vi "lxc.vi"() -> ()   [LabVIEW 2017]
uses:
  <vilib>/Instr/_visa.llb/VISA Flush IO Buffer Mask.ctl
  <vilib>/Instr/_visa.llb/VISA Configure Serial Port (Instr).vi
panel:
  out "波形图表":i32(graph)
  in  "停止":bool
  out "读取缓冲区":string
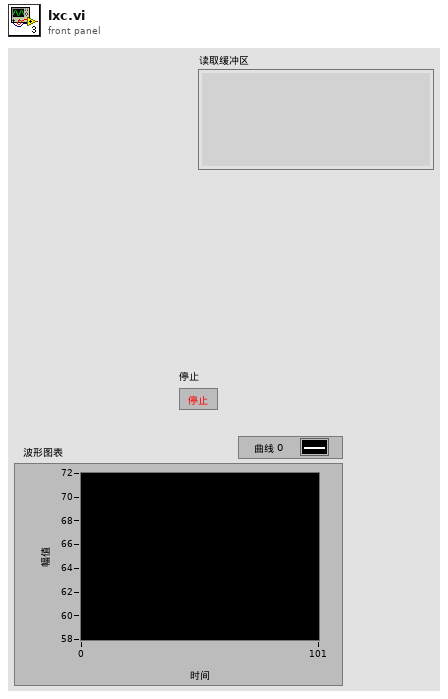
[diagram p1: front panel]
types:
  T1 = typedef "VISA Flush IO Buffer Mask.ctl" = u16
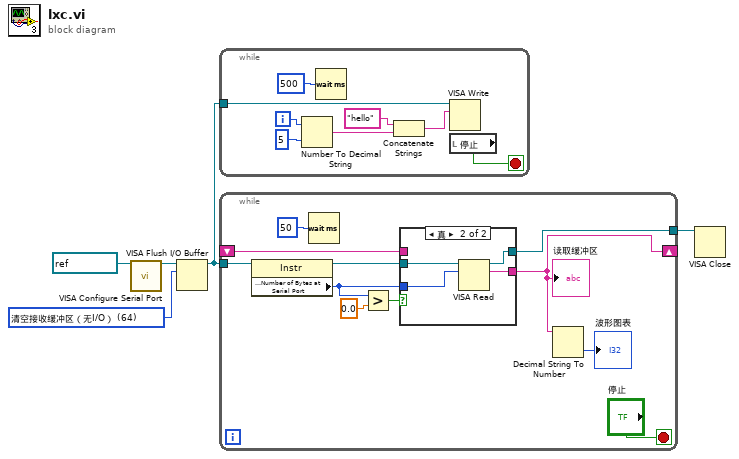
[diagram p0: block diagram]
diagram:
  w3 = T1 64 items=["清空接收缓冲区"=16, "向设备写入传输缓冲区"=32, "清空接收缓冲区（无I/O）"=64, "清空传输缓冲区"=128] ("Mask")
  n1 = call-poly "VISA Configure Serial Port"("VISA resource name"=refnum<visa-resource-name> "COM1") -> ("VISA resource name out"=w1:refnum<visa-resource-name>)  [unwired: 13 in, 1 out]
  n2 = VISA Flush I/O Buffer(VISA resource name=w1, mask (16)=w3) -> (VISA resource name out=w2:refnum<visa-resource-name>)  [unwired: 1 in, 1 out]
  n3 = while {
    tunnel: w2 -> [w13]
    i -> [w10]
    stop <- w11 stop-if-true
    n4 = Number To Decimal String(number=w10, width (-)=i16 5 ("宽度(-)")) -> (decimal integer string=w8:string)
    n5 = Wait (ms)(milliseconds to wait=u32 500 ("等待时间（毫秒）")) -> ()  [unwired: 1 out]
    n6 = Concatenate Strings("hello" ("写入缓冲区"), w8) -> (w7:string)
    n7 = VISA Write(VISA resource name=w13, write buffer=w7) -> ()  [unwired: 1 in, 3 out]
    n8 = local read "停止"() -> (w11:bool)
  }
  n9 = while {
    tunnel: w2 -> [w21]
    shift-right: [w18] -> _
    shift-left: _ -> [w17]
    tunnel: [w14] -> w4
    stop <- "停止" stop-if-true
    n10 = property class="Instr"(reference=w21) -> (reference out=w19:refnum<visa-resource-name>, "Serial Settings:Number of Bytes at Serial Port"=w15:u32)  [unwired: 1 in, 1 out]
    n11 = Wait (ms)(milliseconds to wait=u32 50 ("等待时间（毫秒）")) -> ()  [unwired: 1 out]
    n12 = Greater?(x=w15, y=0.0) -> (0:w16:bool)
    n13 = case shown="真" w16 {
      tunnel: [w25 w29] -> w18
      tunnel: [w25 w28] -> w14
      tunnel: w19 -> [_ w27]
      tunnel: w17 -> [w25 _]
      tunnel: w15 -> [_ w26]
      frame False {
      }
      frame True {
        n14 = VISA Read(VISA resource name=w27, byte count=w26) -> (VISA resource name out=w28:refnum<visa-resource-name>, read buffer=w29:string)  [unwired: 1 in, 2 out]
      }
    }
    "读取缓冲区" <- w18
    n15 = Decimal String To Number(string=w18) -> (number=→"波形图表":i32)  [unwired: 2 in, 1 out]
  }
  n16 = VISA Close(VISA resource name=w4) -> ()  [unwired: 1 in, 1 out]
